vi "Write Unique Name.vi"(8 "error in (no error)":errorcluster, 10 "Unique Name":string, 11 "Component in":refnum<class "Component.lvclass">) -> (0 "error out":errorcluster, 3 "Component out":refnum<class "Component.lvclass">)   [LabVIEW 2017, in "CL_G3_VIComponentBuilder.lvlib" / "Component.lvclass"]
uses:
  Component.lvclass
  Component.lvclass/Component.ctl
  Read Component Config File.vi
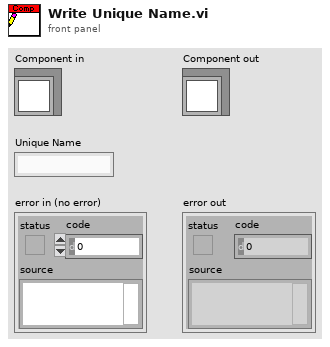
[diagram p1: front panel]
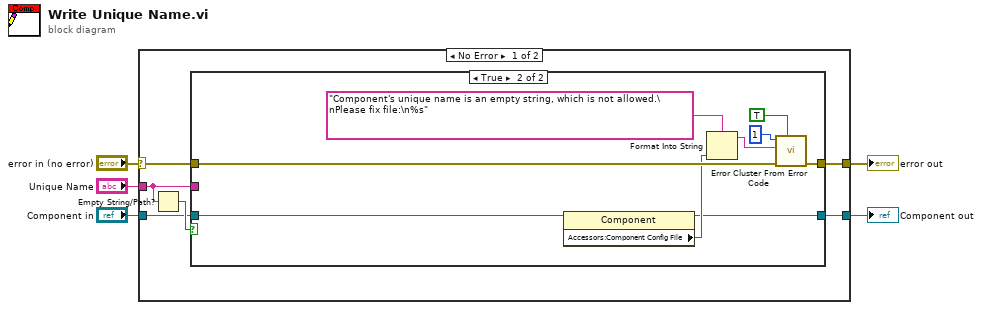
[diagram p0: block diagram]
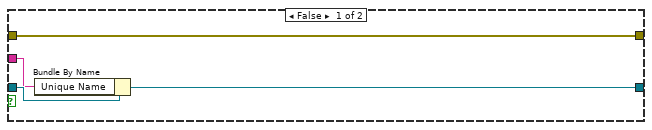
[diagram p2: hidden frame]
diagram:
  n1 = case shown="No Error" "error in (no error)" {
    selector: "error in (no error)" -> [w10 w25]
    tunnel: [w9 w25] -> w4
    tunnel: [w7 w26] -> w2
    tunnel: "Component in" -> [w8 w26]
    tunnel: "Unique Name" -> [w6 _]
    frame No Error {
      n2 = Empty String/Path?(string/path=w6) -> (empty?=w11:bool)
      n3 = case shown="True" w11 {
        tunnel: w10 -> [w15 w24]
        tunnel: [w15 w16] -> w9
        tunnel: w8 -> [w14 w21]
        tunnel: [w13 w18] -> w7
        tunnel: w6 -> [w12 _]
        frame False {
          n4 = Bundle By Name(cluster=w14, "Unique Name"=w12) -> (w13:refnum<class "Component.lvclass">)
        }
        frame True {
          n5 = property class="Component"(reference=w21) -> (reference out=w18:refnum<class "Component.lvclass">, "Accessors:Component Config File"=w19:path)  [unwired: 1 in, 1 out]
          n6 = Format Into String(format string="Component's unique name is an empty string, which is not allowed.\nPlease fix file:\n%s" ("error message (\"\")"), w19) -> (resulting string=w17:string)  [unwired: 2 in, 1 out]
          n7 = call <vilib>:"Error Cluster From Error Code.vi"("show call chain? (False)"=TRUE, "error in (no error)"=w24, "error message (\"\")"=w17, "error code (0)"=1) -> ("error out"=w16:errorcluster)  [unwired: 5 in]
        }
      }
    }
    frame Error {
    }
  }
  "error out" <- w4
  "Component out" <- w2
